vi "DACvals.vi"() -> ()   [LabVIEW 2015]
panel:
  in  "Board 2 / DAC 8":u16=3
  in  "Board 2 / DAC 7":u16=3
  in  "Board 2 / DAC 6":u16=3
  in  "Board 2 / DAC 5":u32=3
  in  "Board 2 / DAC 4":u16=3
  in  "Board 2 / DAC 3":u16=3
  in  "Board 2 / DAC 2":u16=3
  in  "Board 2 / DAC 1":u16=3
  in  "Board 1 / DAC 8":u16=3
  in  "Board 1 / DAC 7":u16=3
  in  "Board 1 / DAC 6":u16=3
  in  "Board 1 / DAC 5":u32=3
  in  "Board 1 / DAC 4":u16=3
  in  "Board 1 / DAC 3":u16=3
  in  "Board 1 / DAC 2":u16=3
  in  "Board 1 / DAC 1":u16=3
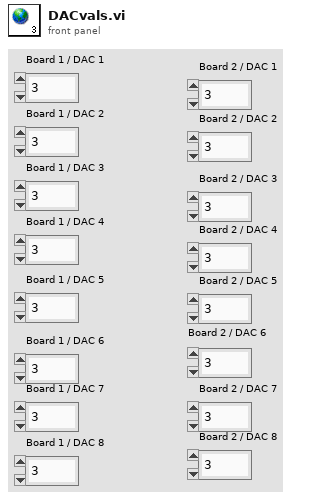
[diagram p1: front panel]
diagram:
